vi "genGrooveV2.vi"() -> ()   [LabVIEW 2016]
uses:
  <vilib>/Math Plots/3D Math Plots/3D Scatter/3D Scatter XCtrl/3D Scatter.xctl
  <vilib>/Analysis/1siggen.llb/Ramp Pattern by Samples.vi
  Subsystems/Global Variables.vi
  <vilib>/Math Plots/3D Math Plots/3D Scatter/3D Scatter Datatype/Public/Plot Helper (Vector).vi
  <vilib>/Math Plots/3D Math Plots/3D Scatter/3D Scatter Datatype/3D Scatter Datatype.lvclass
  <vilib>/gmath/NI_Gmath.lvlib
  <vilib>/Analysis/NI_AALBase.lvlib
panel:
  in  "Eye":dbl
  in  "trial_no":dbl
  in  "offset":dbl
  out "size(s)":i32
  out "zVisTraj":dbl[](array[numeric]) format="%_6g"
  out "yVisTraj":dbl[](array[numeric]) format="%_6g"
  out "xVisTraj":dbl[](array[numeric]) format="%_6g"
  out "Groove Plot":refnum<class "3D Plot Datatype.lvclass">[](xcontrol)
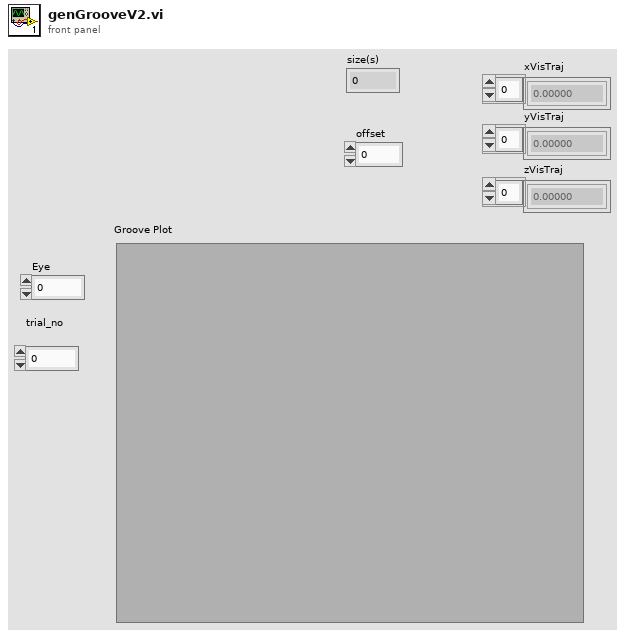
[diagram p1: front panel]
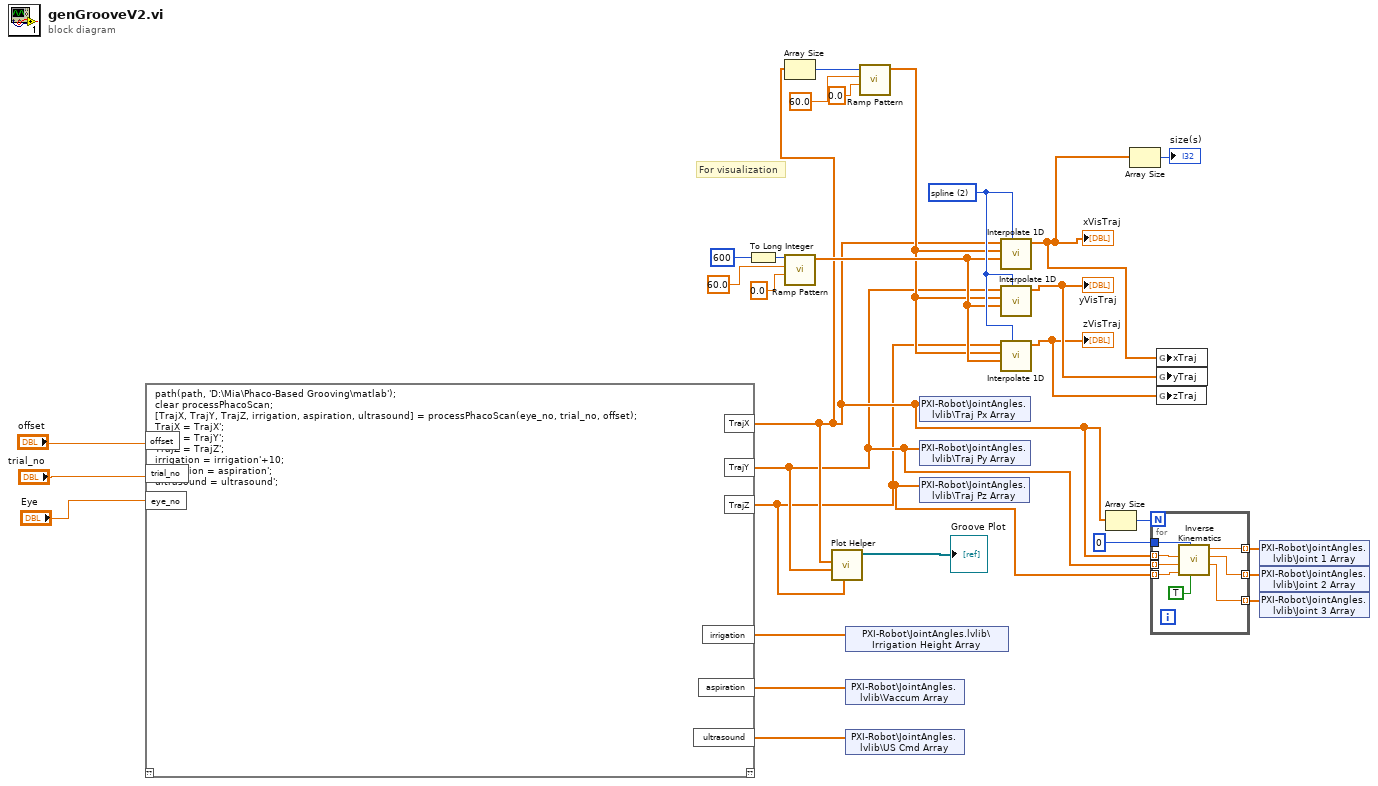
[diagram p0: block diagram]
diagram:
  w28 = 2 items=["nearest", "linear", "spline", "cubic Hermite", "Lagrange"] ("method")
  # "For visualization"
  n1 = script code="path(path, 'D:\\Mia\\Phaco-Based Grooving\\matlab'); \nclear processPhacoScan;\n[TrajX, TrajY, TrajZ, irrigation, aspiration, ultrasound] = processPhacoScan(eye_no, trial_no, offset);\nTrajX = TrajX'; \nTrajY = TrajY'; \nTrajZ = TrajZ'; \nirrigation = irrigation'+10;\naspiration = aspiration';\nultrasound = ultrasound';"("offset"="offset", "trial_no"="trial_no", "eye_no"="Eye") -> ("TrajX"=w5:dbl[], "TrajY"=w4:dbl[], "TrajZ"=w3:dbl[], "irrigation"=w13:dbl[], "aspiration"=w1:dbl[], "ultrasound"=w14:dbl[])  [unwired: 1 in, 1 out]
  n2 = To Long Integer(number=600) -> (32bit integer=w27:i32)
  n3 = Array Size(array=w5) -> (size(s)=w21:i32)
  n4 = call-poly <vilib>:"Ramp Pattern.vi"("start"=0.0, "end"=60.0, "samples"=w27) -> ("Ramp Pattern"=w25:dbl[])  [unwired: 7 in, 1 out]
  n5 = call-poly <vilib>:"Plot Helper.vi"("z vector"=w3, "y vector"=w4, "x vector"=w5) -> ("3D Plot lvclass Array out"=→"Groove Plot":refnum<class "3D Plot Datatype.lvclass">[])  [unwired: 3 in, 5 out]
  n6 = shared-variable "PXI-Robot\\JointAngles.lvlib\\Irrigation Height Array"(w13) -> ()  [unwired: 1 in, 1 out]
  n7 = shared-variable "PXI-Robot\\JointAngles.lvlib\\Vaccum Array"(w1) -> ()  [unwired: 1 in, 1 out]
  n8 = shared-variable "PXI-Robot\\JointAngles.lvlib\\US Cmd Array"(w14) -> ()  [unwired: 1 in, 1 out]
  n9 = call-poly <vilib>:"Ramp Pattern.vi"("start"=0.0, "end"=60.0, "samples"=w21) -> ("Ramp Pattern"=w20:dbl[])  [unwired: 7 in, 1 out]
  n10 = shared-variable "PXI-Robot\\JointAngles.lvlib\\Traj Px Array"(w5) -> ()  [unwired: 1 in, 1 out]
  n11 = shared-variable "PXI-Robot\\JointAngles.lvlib\\Traj Py Array"(w4) -> ()  [unwired: 1 in, 1 out]
  n12 = shared-variable "PXI-Robot\\JointAngles.lvlib\\Traj Pz Array"(w3) -> ()  [unwired: 1 in, 1 out]
  n13 = call <vilib>:"Interpolate 1D.vi"("method"=w28, "xi"=w25, "X"=w20, "Y"=w5) -> ("yi"=w12:dbl[])  [unwired: 5 in, 2 out]
  "xVisTraj" <- w12
  n14 = call <vilib>:"Interpolate 1D.vi"("method"=w28, "xi"=w25, "X"=w20, "Y"=w4) -> ("yi"=w11:dbl[])  [unwired: 5 in, 2 out]
  "yVisTraj" <- w11
  n15 = call <vilib>:"Interpolate 1D.vi"("method"=w28, "xi"=w25, "X"=w20, "Y"=w3) -> ("yi"=w10:dbl[])  [unwired: 5 in, 2 out]
  "zVisTraj" <- w10
  n16 = Array Size(array=w5) -> (size(s)=w9:i32)
  n17 = Array Size(array=w12) -> (size(s)=→"size(s)":i32)
  n18 = for {
    N: w9 -> [_]
    tunnel: 0 ("Arm ID Ind") -> [w33]
    tunnel: w5 -> [w37] mode=indexing
    tunnel: w4 -> [w36] mode=indexing
    tunnel: w3 -> [w35] mode=indexing
    tunnel: [w32] -> w8 mode=indexing
    tunnel: [w31] -> w7 mode=indexing
    tunnel: [w30] -> w6 mode=indexing
    n19 = call "Inverse Kinematics.vi"("isToolTipInsideEye"=TRUE, "armID"=w33, "z"=w35, "y"=w36, "x"=w37) -> ("j3"=w30:dbl, "j2"=w31:dbl, "j1"=w32:dbl)  [unwired: 3 in, 1 out]
  }
  n20 = global write "Global Variables.vi" "xTraj"(w12) -> ()
  n21 = global write "Global Variables.vi" "yTraj"(w11) -> ()
  n22 = global write "Global Variables.vi" "zTraj"(w10) -> ()
  n23 = shared-variable "PXI-Robot\\JointAngles.lvlib\\Joint 1 Array"(w8) -> ()  [unwired: 1 in, 1 out]
  n24 = shared-variable "PXI-Robot\\JointAngles.lvlib\\Joint 2 Array"(w7) -> ()  [unwired: 1 in, 1 out]
  n25 = shared-variable "PXI-Robot\\JointAngles.lvlib\\Joint 3 Array"(w6) -> ()  [unwired: 1 in, 1 out]
